vi "Make Center String.vi"(8 "error in (no error)":errorcluster, 10 "Location string":string) -> (0 "error out":errorcluster, 2 "Center string":string)   [LabVIEW 2012]
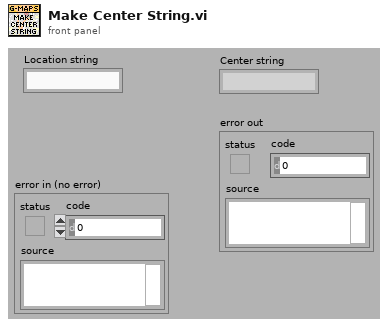
[diagram p1: front panel]
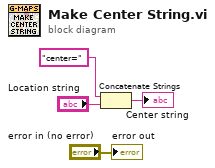
[diagram p0: block diagram]
diagram:
  n1 = Concatenate Strings("center=" ("URL"), "Location string") -> (→"Center string":string)
  "error out" <- "error in (no error)"
